vi "Equals.vi"(1 "comparable b":refnum<class "Equal Comparable.lvclass">, 2 "comparable a":refnum<class "Equal Comparable.lvclass">, 3 "Equals Functor":refnum<class "Equal Functor.lvclass">) -> (0 "equal?":bool)   [LabVIEW 2020, in "Equal Functor.lvclass"]
doc: "Returns whether <b>Comparable 1</b> is less than, equal to, or greater than <b>Comparable 2</b>."
uses:
  <vilib>/Comparison/Equal/Equal Functor/Equal Functor.lvclass
  <vilib>/Comparison/Equal/Equal Comparable/Equal Comparable.lvclass
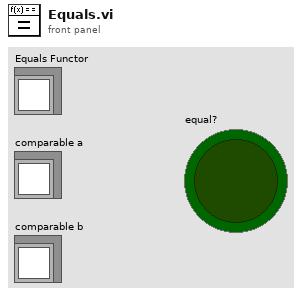
[diagram p1: front panel]
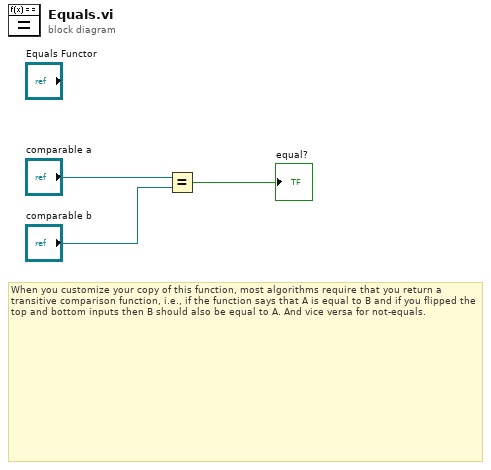
[diagram p0: block diagram]
diagram:
  # "When you customize your copy of this function, most algorithms require that you return a transitive comparison function, i.e., if the function says that A is equal to B and if you flipped the top and bottom inputs then B should also be equal to A. And vice versa for not-equals."
  n1 = Equal?(x="comparable a", y="comparable b") -> (x = y?=→"equal?":bool)
